vi "Filter Selection.vi"(4 "Ext. Selection":i32[](array[numeric])) -> (1 "Filtered Selection":i32[](array[numeric]))   [LabVIEW 2015, in "LV Image Editor Framework.lvlib" / "Image Editor Handler.lvclass"]
uses:
  Image Editor Handler.lvclass
panel:
  out "error out":errorcluster
  in  "error in (no error)":errorcluster
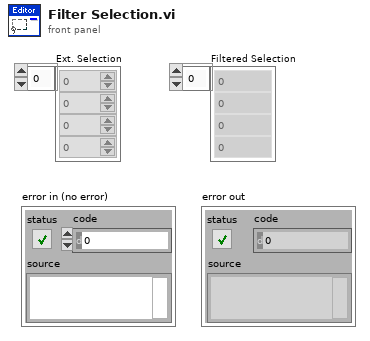
[diagram p1: front panel]
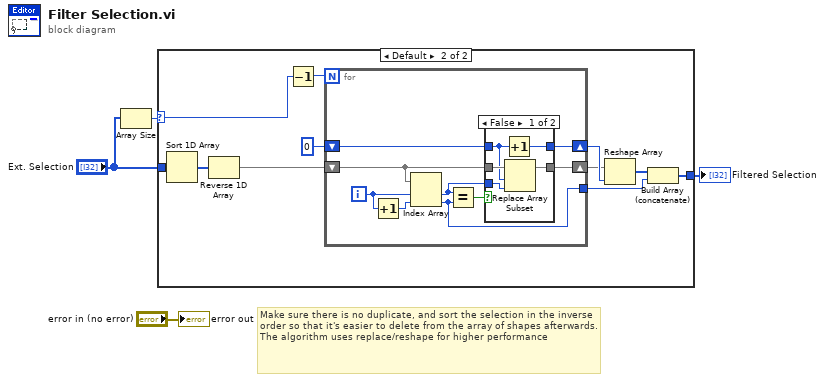
[diagram p0: block diagram]
diagram:
  # "Make sure there is no duplicate, and sort the selection in the inverse order so that it's easier to delete from the array of shapes afterwards.\nThe algorithm uses replace/reshape for higher performance"
  n1 = Array Size(array="Ext. Selection") -> (size(s)=w1:i32)
  n2 = case shown="Default" w1 {
    selector: w1 -> [_ w6]
    tunnel: "Ext. Selection" -> [w5 w8]
    tunnel: [w5 w7] -> w3
    frame 0, 1 {
    }
    frame Default {
      n3 = Sort 1D Array(array=w8) -> (sorted array=w10:i32[])
      n4 = Reverse 1D Array(array=w10) -> (reversed array=w9:i32[])
      n5 = Decrement(x=w6) -> (x-1=w16:i32)
      n6 = for {
        N: w16 -> [_]
        shift-right: [w23] -> w14
        shift-left: 0 -> [w21]
        shift-right: [w22] -> w13
        shift-left: w9 -> [w24]
        tunnel: [w17] -> w11
        i -> [w18]
        n7 = Increment(x=w18) -> (x+1=w20:i32)
        n8 = Index Array(array=w24, index #1=w18, index #2=w20) -> (element #1=w19:i32, element #2=w17:i32)
        n9 = Equal?(x=w19, y=w17) -> (x = y?=w25:bool)
        n10 = case shown="False" w25 {
          tunnel: w24 -> [w30 w32]
          tunnel: w21 -> [w27 w31]
          tunnel: [w28 w31] -> w23
          tunnel: [w29 w32] -> w22
          tunnel: w19 -> [w26 _]
          frame False {
            n11 = Increment(x=w27) -> (x+1=w28:i32)
            n12 = Replace Array Subset(array=w30, new element=w26, index=w27) -> (w29:i32[])
          }
          frame True {
          }
        }
      }
      n13 = Reshape Array(w13, w14) -> (w12:i32[])
      n14 = Build Array (concatenate)(w12, w11) -> (w7:i32[])
    }
  }
  "Filtered Selection" <- w3
  "error out" <- "error in (no error)"
